vi "gyro_check_1.vi"() -> (2 "has the drone landed?":bool)   [LabVIEW 2019]
uses:
  <vilib>/myRIO/Instrument Drivers/Onboard Devices/Accelerometer/typedefs/Accelerometer Reference.ctl
  <vilib>/myRIO/Common/Instrument Driver Framework/Utilities/typedefs/myRIO Generic Hardware Reference.ctl
  <vilib>/myRIO/Common/Instrument Driver Framework/Utilities/typedefs/Hardware Version Enum.ctl
  <vilib>/myRIO/Common/Instrument Driver Framework/Utilities/typedefs/myRIO v1.0 Reference.ctl
  <vilib>/myRIO/Common/Instrument Driver Framework/Utilities/typedefs/Generic FPGA Reference.ctl
  <vilib>/myRIO/Common/Instrument Driver Framework/myRIO v1.0/Accelerometer/typedefs/Accelerometer Channels List.ctl
  <vilib>/myRIO/Common/Instrument Driver Framework/myRIO v1.0/Accelerometer/typedefs/Accelerometer Channels Enum.ctl
  <vilib>/userdefined/High Color/nirio_resource_hc.ctl
  <vilib>/myRIO/Instrument Drivers/Onboard IO/DIO/typedefs/DIO Reference.ctl
  <vilib>/myRIO/Common/Instrument Driver Framework/myRIO v1.0/DIO/typedefs/DIO Channels List.ctl
  <vilib>/myRIO/Common/Instrument Driver Framework/myRIO v1.0/DIO/typedefs/DIO Channels Enum.ctl
  <vilib>/myRIO/Common/Instrument Driver Framework/Utilities/vis/Is FPGA Ref Available.vi
  <vilib>/myRIO/Common/Instrument Driver Framework/myRIO v1.0/Accelerometer/vis/myRIO v1.1 Open Accelerometer.vi
  <vilib>/myRIO/Instrument Drivers/Onboard Devices/Accelerometer/vis/Read.vi
  <vilib>/myRIO/Common/Instrument Driver Framework/myRIO v1.0/DIO/vis/myRIO v1.1 Open DIO.vi
  <vilib>/myRIO/Instrument Drivers/Onboard IO/DIO/vis/Write.vi
  <vilib>/myRIO/Common/Instrument Driver Framework/Utilities/vis/Validate Channels.vi
  <vilib>/myRIO/Common/Instrument Driver Framework/myRIO v1.0/Accelerometer/vis/myRIO v1.0 Reserve Accelerometer.vi
  <vilib>/myRIO/Common/Instrument Driver Framework/myRIO v1.0/DIO/vis/myRIO v1.0 Reserve DIO.vi
  <vilib>/myRIO/Common/Instrument Driver Framework/myRIO v1.0/Resource Manager/vis/myRIO v1.0 Reserve Channel List.vi
  <vilib>/myRIO/Common/Instrument Driver Framework/myRIO v1.0/Accelerometer/vis/myRIO v1.0 Build MUX Configuration Accelerometer.vi
  <vilib>/myRIO/Common/Instrument Driver Framework/myRIO v1.0/DIO/vis/myRIO v1.0 Build MUX Configuration DIO.vi
  <vilib>/myRIO/Common/Instrument Driver Framework/myRIO v1.0/Resource Manager/vis/myRIO v1.0 Reserve Channel.vi
  <vilib>/myRIO/Common/Instrument Driver Framework/myRIO v1.0/Resource Manager/vis/myRIO v1.0 Unreserve Channel.vi
  <vilib>/myRIO/Common/Instrument Driver Framework/myRIO v1.0/Resource Manager/vis/myRIO v1.0 Create Configuration List.vi
  <vilib>/myRIO/Common/Instrument Driver Framework/myRIO v1.0/Resource Manager/vis/myRIO v1.0 Build Mutex Name.vi
  <vilib>/Utility/VariantDataType/GetNumericInfo.vi
  <vilib>/Utility/error.llb/Error Cluster From Error Code.vi
  <vilib>/myRIO/Common/Instrument Driver Framework/myRIO v1.0/myRIO v1.1 Open.vi
  <vilib>/myRIO/Common/Instrument Driver Framework/myRIO v1.0/Accelerometer/vis/myRIO v1.0 Get Scaling Constant Accelerometer.vi
  <vilib>/myRIO/Common/Instrument Driver Framework/Utilities/vis/IO Manager.vi
  <vilib>/myRIO/Common/Instrument Driver Framework/Utilities/vis/Configuration Manager.vi
  <vilib>/myRIO/Common/Instrument Driver Framework/myRIO v1.0/myRIO v1.0 Close.vi
  <vilib>/myRIO/Common/Instrument Driver Framework/myRIO v1.0/Accelerometer/vis/myRIO v1.0 Read Accelerometer.vi
  <vilib>/myRIO/Common/Instrument Driver Framework/myRIO v1.0/Resource Manager/vis/myRIO v1.0 Configure IO.vi
  <vilib>/myRIO/Common/Instrument Driver Framework/myRIO v1.0/DIO/vis/myRIO v1.0 Write DIO.vi
  <vilib>/Utility/file.llb/Write Delimited Spreadsheet (DBL).vi
  <vilib>/myRIO/Express VI/Onboard Devices/Accelerometer/Accelerometer Express VI.xnode
  <vilib>/myRIO/Instrument Drivers/Onboard Devices/Accelerometer/vis/myRIO Accelerometer Open.xnode
  <vilib>/myRIO/Express VI/Onboard Devices/LED/LED Express VI.xnode
  <vilib>/myRIO/Instrument Drivers/Onboard IO/DIO/vis/myRIO DIO Open.xnode
  <vilib>/myRIO/Instrument Drivers/Onboard Devices/Accelerometer/Accelerometer.lvlib
  <vilib>/myRIO/Instrument Drivers/Onboard IO/DIO/DIO.lvlib
panel:
  out "Distance of height sensor from the ground":dbl
  out "z-axis acc":dbl
  out "y-axis acc":dbl
  out "x-axis acc":dbl
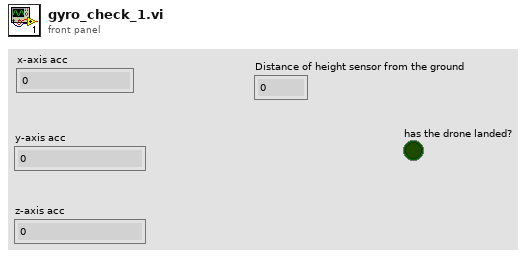
[diagram p1: front panel]
types:
  T1 = typedef "DIO.lvlib/DIO Reference.ctl" = cluster{"myRIO Reference":T2, "DIO Channels List":T6}
  T2 = typedef "myRIO Generic Hardware Reference.ctl" = cluster{"myRIO Model":T3, "myRIO Hardware Reference":T4}
  T3 = typedef "Hardware Version Enum.ctl" = enum16{"Unknown", "myRIO-1900", "myRIO-1950", "roboRIO", "NI ELVIS RIO CM", "ELVIS III"}
  T4 = typedef "myRIO v1.0 Reference.ctl" = cluster{"Generic FPGA Reference":T5, "Allow multiple opens":bool}
  T5 = typedef "Generic FPGA Reference.ctl" = refnum<k20>
  T6 = typedef "DIO Channels List.ctl" = T7[]
  T7 = typedef "DIO Channels Enum.ctl" = enum16{"Not Connected", "C/DIO0", "C/DIO1", "C/DIO2", "C/DIO3", "C/DIO4", "C/DIO5", "C/DIO6", "C/DIO7", "A/DIO0", "A/DIO1", "A/DIO2", "A/DIO3", "A/DIO4", "A/DIO5", "A/DIO6", "A/DIO7", "A/DIO8", "A/DIO9", "A/DIO10", "A/DIO11", "A/DIO12", "A/DIO13", "A/DIO14", "A/DIO15", "A/DIO16", "A/DIO17", "A/DIO18", "A/DIO19", "B/DIO0", "B/DIO1", "B/DIO2", "B/DIO3", "B/DIO4", "B/DIO5", "B/DIO6", "B/DIO7", "B/DIO8", "B/DIO9", "B/DIO10", "B/DIO11", "B/DIO12", "B/DIO13", "B/DIO14", "B/DIO15", "B/DIO16", "B/DIO17", "B/DIO18", "B/DIO19", "LED0", "LED1", "LED2", "LED3", "Button0", "DIO/DIO0", "DIO/DIO1", "DIO/DIO2", "DIO/DIO3", "DIO/DIO4", "DIO/DIO5", "DIO/DIO6", "DIO/DIO7", "DIO/DIO8", "DIO/DIO9", "SPI/CS0", "SPI/CS1", "SPI/CS2", "SPI/CS3", "LED RADIO (Green)", "LED RADIO (Red)", "LED COMM (Green)", "LED COMM (Red)", "LED MODE (Green)", "LED MODE (Red)"}
  T8 = typedef "nirio_resource_hc.ctl" = tag
  T9 = typedef "Accelerometer.lvlib/Accelerometer Reference.ctl" = cluster{"myRIO Reference":T2, "Accelerometer Channels List":T10, "LSB Weight":dbl}
  T10 = typedef "Accelerometer Channels List.ctl" = T11[]
  T11 = typedef "Accelerometer Channels Enum.ctl" = enum16{"Not Connected", "X-Axis", "Y-Axis", "Z-Axis"}
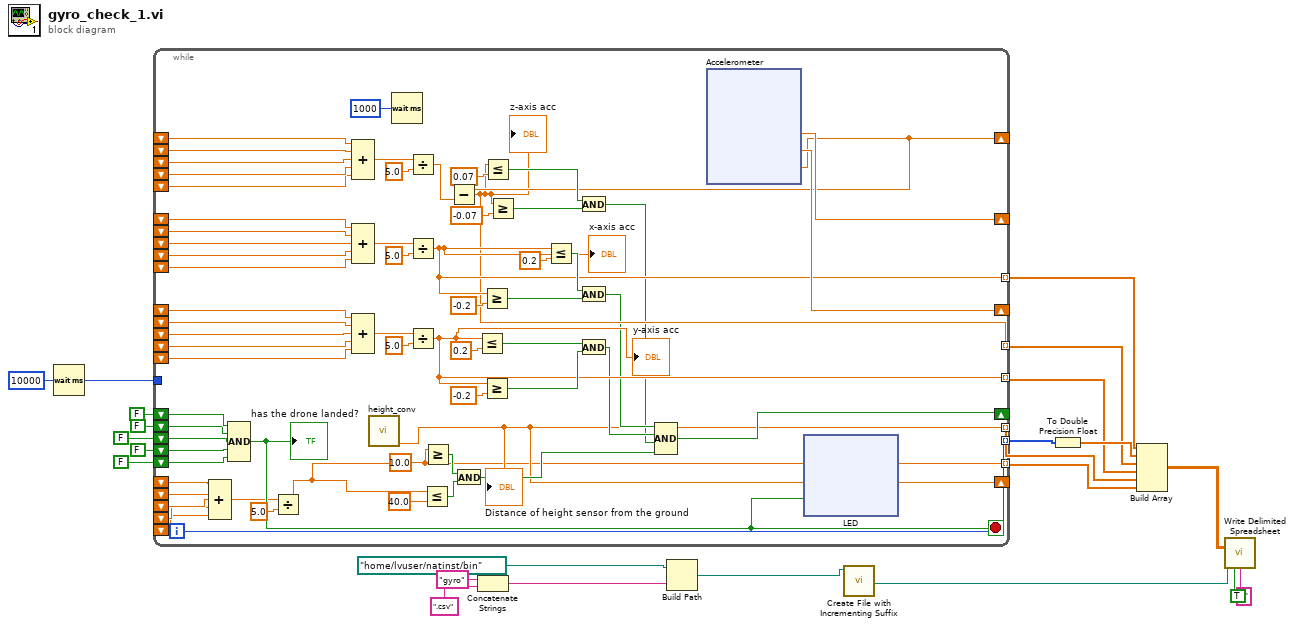
[diagram p0: block diagram]
diagram:
  n1 = Wait (ms)(milliseconds to wait=u32 10000) -> (millisecond timer value=w23:u32)
  n2 = while {
    shift-right: [w89] -> _
    shift-left: _ -> [w74]
    shift-right: [w88] -> _
    shift-left: _ -> [w66]
    shift-right: [w49] -> _
    shift-left: _ -> [w59]
    shift-left: _ -> [w73]
    shift-left: _ -> [w72]
    shift-left: _ -> [w71]
    shift-left: _ -> [w70]
    shift-left: _ -> [w65]
    shift-left: _ -> [w64]
    shift-left: _ -> [w63]
    shift-left: _ -> [w62]
    shift-left: _ -> [w58]
    shift-left: _ -> [w57]
    shift-left: _ -> [w56]
    shift-left: _ -> [w55]
    shift-right: [w33] -> _
    shift-left: FALSE -> [w47]
    shift-left: FALSE -> [w46]
    shift-left: FALSE -> [w45]
    shift-left: FALSE -> [w44]
    shift-left: FALSE -> [w43]
    tunnel: w23 -> [_]
    tunnel: [w41] -> w14 mode=indexing
    tunnel: [w40] -> w15 mode=indexing
    tunnel: [w39] -> w9 mode=indexing
    tunnel: [w38] -> w8 mode=indexing
    tunnel: [w32] -> w7 mode=indexing
    shift-right: [w32] -> _
    shift-left: _ -> [w31]
    shift-left: _ -> [w30]
    shift-left: _ -> [w29]
    shift-left: _ -> [w28]
    shift-left: _ -> [w27]
    tunnel: [w24] -> w6 mode=indexing
    i -> [w40]
    stop <- w42 stop-if-true
    n3 = Compound Arithmetic op=ADD(w31, w30, w29, w28, w27) -> (w25:dbl)
    n4 = Compound Arithmetic op=AND(w47, w46, w45, w44, w43) -> (w42:bool)
    "has the drone landed?" <- w42
    n5 = Divide(x=w25, y=5.0) -> (x/y=w24:dbl)
    n6 = Compound Arithmetic op=ADD(w59, w58, w57, w56, w55) -> (w61:dbl)
    n7 = Compound Arithmetic op=ADD(w74, w73, w72, w71, w70) -> (w54:dbl)
    n8 = Compound Arithmetic op=ADD(w66, w65, w64, w63, w62) -> (w67:dbl)
    n9 = call "height_conv.vi"() -> ("Distance of sensor from the ground"=w32:dbl)  [unwired: 11 in]
    "Distance of height sensor from the ground" <- w32
    n10 = Wait (ms)(milliseconds to wait=u32 1000) -> ()  [unwired: 1 out]
    n11 = Divide(x=w61, y=5.0) -> (x/y=w48:dbl)
    n12 = Divide(x=w54, y=5.0) -> (x/y=w41:dbl)
    "x-axis acc" <- w41
    n13 = Divide(x=w67, y=5.0) -> (x/y=w38:dbl)
    "y-axis acc" <- w38
    n14 = Less Or Equal?(x=w24, y=40.0) -> (x <= y?=w51:bool)
    n15 = Greater Or Equal?(x=w24, y=10.0) -> (x >= y?=w50:bool)
    n16 = And(x=w50, y=w51) -> (x .and. y?=w37:bool)
    n17 = Less Or Equal?(x=w38, y=0.2) -> (x <= y?=w79:bool)
    n18 = Greater Or Equal?(x=w41, y=-0.2) -> (x >= y?=w80:bool)
    n19 = Greater Or Equal?(x=w38, y=-0.2) -> (x >= y?=w78:bool)
    n20 = Less Or Equal?(x=w41, y=0.2) -> (x <= y?=w81:bool)
    n21 = And(x=w81, y=w80) -> (x .and. y?=w35:bool)
    n22 = And(x=w79, y=w78) -> (x .and. y?=w36:bool)
    n23 = xnode "Accelerometer"() -> ("X-Axis"=w89:dbl, "Y-Axis"=w88:dbl, "Z-Axis"=w49:dbl)  [unwired: 1 in, 1 out]
    n24 = Subtract(x=w49, y=w48) -> (x-y=w39:dbl)
    "z-axis acc" <- w39
    n25 = Less Or Equal?(x=w39, y=0.07) -> (x <= y?=w77:bool)
    n26 = Greater Or Equal?(x=w39, y=-0.07) -> (x >= y?=w76:bool)
    n27 = And(x=w77, y=w76) -> (x .and. y?=w34:bool)
    n28 = Compound Arithmetic op=AND(w35, w36, w34, w37) -> (w33:bool)
    n29 = xnode "LED"("LED3"=w42) -> ()  [unwired: 1 in, 1 out]
  }
  n30 = Concatenate Strings("gyro" ("string"), ".csv" ("string")) -> (w19:string)
  n31 = Build Path(base path=path "/home/lvuser/natinst/bin", name or relative path=w19) -> (appended path=w11:path)
  n32 = call <vilib>:"Create File with Incrementing Suffix.vi"("file path"=w11) -> ("actual path"=w10:path)  [unwired: 8 in, 2 out]
  n33 = To Double Precision Float(number=w15) -> (double precision float=w13:dbl[])
  n34 = Build Array(w14, w13, w9, w8, w7, w6) -> (w12:dbl[][])
  n35 = call-poly <vilib>:"Write Delimited Spreadsheet.vi"("file path (dialog if empty)"=w10, "2D data"=w12, "transpose? (no:F)"=TRUE, "delimiter (\\t)"="," ("delimiter (\\t)")) -> ()  [unwired: 10 in, 2 out]
